vi "action.vi"(0 "HGF_FGV_Action":refnum<class "HGF_FGV_Action.lvclass">, 2 "Objects":refnum<class>[](array[class]), 5 "error in (no error)":errorcluster) -> (14 "dup HGF_FGV_Action":refnum<class "HGF_FGV_Action.lvclass">, 16 "dup Objects":refnum<class>[](array[class]), 19 "error out":errorcluster)   [LabVIEW 2012, in "HGF_FGV.lvlib" / "HGF_FGV_Action.lvclass"]
doc: "This is a dynamic dispatch VI. It must be overwritten by child classes.to implement the concrete action."
uses:
  HGF_FGV_Action.lvclass
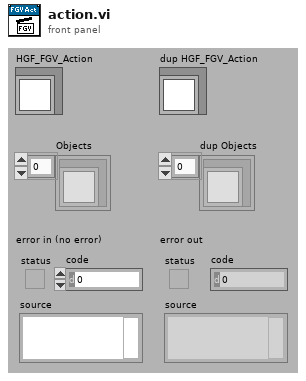
[diagram p1: front panel]
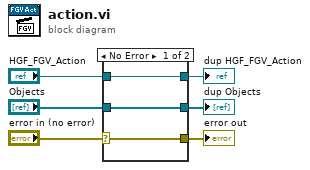
[diagram p0: block diagram]
diagram:
  n1 = case shown="No Error" "error in (no error)" {
    selector: "error in (no error)" -> [w8 w12]
    tunnel: [w8 w12] -> w5
    tunnel: [w9 w11] -> w3
    tunnel: "HGF_FGV_Action" -> [w9 w11]
    tunnel: [w7 w10] -> w2
    tunnel: "Objects" -> [w7 w10]
    frame No Error {
    }
    frame Error {
    }
  }
  "error out" <- w5
  "dup HGF_FGV_Action" <- w3
  "dup Objects" <- w2
